vi "Read POS.vi"(8 "error in (no error)":errorcluster, 11 "SMSD in":refnum<class "SMSD.lvclass">) -> (0 "error out":errorcluster, 2 "POS":i32, 3 "SMSD out":refnum<class "SMSD.lvclass">)   [LabVIEW 2021, in "SMSD.lvclass"]
uses:
  SMSD.lvclass
  SMSD.lvclass/SMSD.ctl
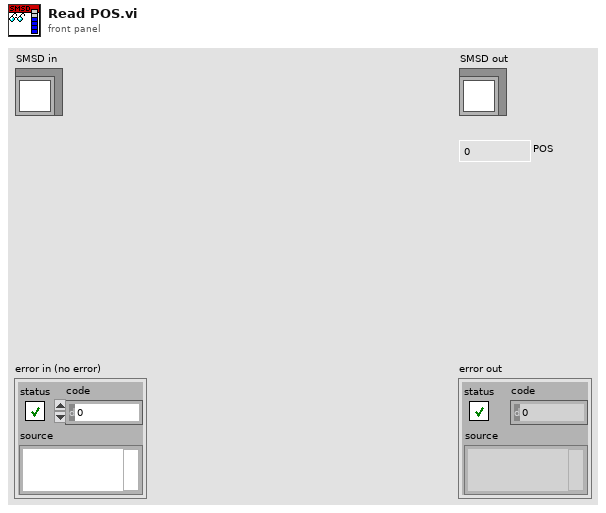
[diagram p1: front panel]
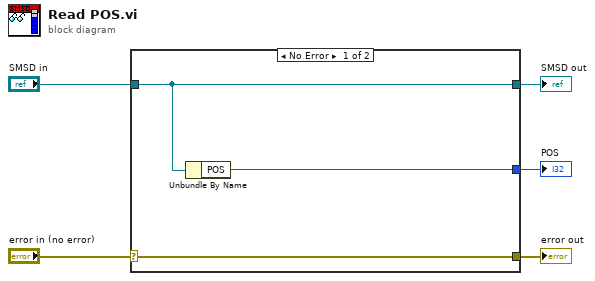
[diagram p0: block diagram]
diagram:
  n1 = case shown="No Error" "error in (no error)" {
    selector: "error in (no error)" -> [w8 w9]
    tunnel: [w8 w9] -> w4
    tunnel: [w7 w10] -> w2
    tunnel: "SMSD in" -> [w7 w10]
    tunnel: [w6 _] -> w1
    frame No Error {
      n2 = Unbundle By Name(w7) -> ("POS"=w6:i32)
    }
    frame Error {
    }
  }
  "error out" <- w4
  "SMSD out" <- w2
  "POS" <- w1
